vi "subtract.vi"(8 "error in (no error)":errorcluster, 11 "params":refnum<class "JSON Null.lvclass">) -> (0 "error out":errorcluster, 3 "data":refnum<class "JSON Null.lvclass">)   [LabVIEW 2015]
uses:
  <vilib>/National Instruments/JSON Support for LabVIEW/JSON Data Classes/JSON Datatype/JSON Null.lvclass
  <vilib>/National Instruments/JSON Support for LabVIEW/JSON Data Classes/JSON Helper/To More Specific Type (Array).vi
  <vilib>/National Instruments/JSON Support for LabVIEW/JSON Data Classes/JSON Array/Index Array (Numeric Value).vi
  <vilib>/National Instruments/JSON Support for LabVIEW/JSON Data Classes/JSON Numeric/New JSON Numeric.vi
  <vilib>/National Instruments/JSON Support for LabVIEW/JSON Data Classes/JSON Array/JSON Array.lvclass
  <vilib>/National Instruments/JSON Support for LabVIEW/JSON Data Classes/JSON Helper/JSON Helper.lvclass
  <vilib>/National Instruments/JSON Support for LabVIEW/JSON Data Classes/JSON Numeric/JSON Numeric.lvclass
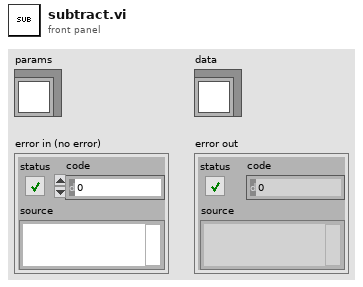
[diagram p1: front panel]
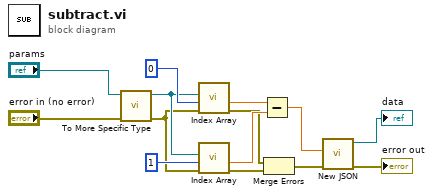
[diagram p0: block diagram]
diagram:
  n1 = call-poly <vilib>:"To More Specific Type.vi"("error in (no error)"="error in (no error)", "JSON Datatype in"="params") -> ("error out"=w5:errorcluster, "JSON Datatype out"=w11:refnum<class "JSON Array.lvclass">)  [unwired: 8 in]
  n2 = call-poly <vilib>:"Index Array.vi"("error in (no error)"=w5, "index"=0, "JSON Array in"=w11) -> ("error out"=w4:errorcluster, "Numeric"=w10:dbl)  [unwired: 7 in]
  n3 = call-poly <vilib>:"Index Array.vi"("error in (no error)"=w5, "index"=1, "JSON Array in"=w11) -> ("error out"=w3:errorcluster, "Numeric"=w9:dbl)  [unwired: 7 in]
  n4 = Subtract(x=w10, y=w9) -> (x-y=w8:dbl)
  n5 = Merge Errors(w4, w3) -> (w2:errorcluster)
  n6 = call-poly <vilib>:"New JSON.vi"("error in (no error)"=w2, "value"=w8) -> ("error out"=→"error out":errorcluster, "JSON String out"=→"data":refnum<class "JSON Numeric.lvclass">)  [unwired: 8 in]
